vi "displayPlainText.vi"(6 "Justification":enum16{"Left", "Center", "Right"}(ring), 8 "error in (no error)":errorcluster, 9 "Font Size":u8=70, 10 "Text In":string, 11 "TextDisplay Class in":refnum<class "TextDisplay Class.lvclass">) -> (0 "error out":errorcluster, 3 "TextDisplay Class out":refnum<class "TextDisplay Class.lvclass">)   [LabVIEW 2020, in "TextDisplay Class.lvclass"]
uses:
  TextDisplay Class.lvclass
  TextDisplay Class.lvclass/TextDisplay Class.ctl
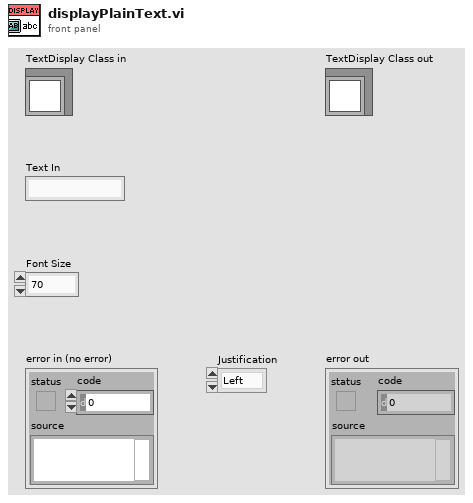
[diagram p1: front panel]
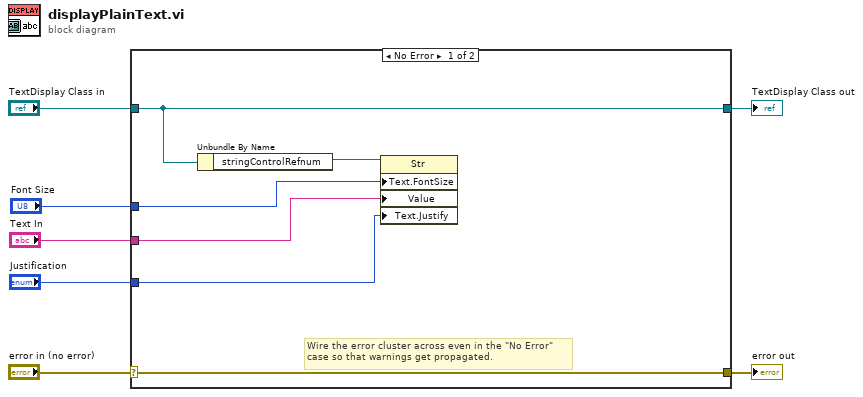
[diagram p0: block diagram]
diagram:
  n1 = case shown="No Error" "error in (no error)" {
    selector: "error in (no error)" -> [w13 w15]
    tunnel: [w13 w15] -> w6
    tunnel: [w12 w14] -> w4
    tunnel: "TextDisplay Class in" -> [w12 w14]
    tunnel: "Text In" -> [w10 _]
    tunnel: "Font Size" -> [w9 _]
    tunnel: "Justification" -> [w8 _]
    frame No Error {
      # "Wire the error cluster across even in the \"No Error\"\ncase so that warnings get propagated."
      n2 = Unbundle By Name(w12) -> ("stringControlRefnum"=w11:refnum<vi>)
      n3 = property class="Str"(reference=w11, "Text.FontSize"=w9, "Value"=w10, "Text.Justify"=w8) -> ()  [unwired: 1 in, 2 out]
    }
    frame Error {
    }
  }
  "error out" <- w6
  "TextDisplay Class out" <- w4
